vi "fit function - hyperbola.vi"(3 "output control":T1, 4 "data":T2, 5 "X":dbl[](array[numeric]), 6 "a":dbl[](array[numeric])) -> (0 "error out":errorcluster, 1 "f'(X,a)":dbl[][](array[numeric]), 2 "f(X,a)":dbl[](array[numeric]))   [LabVIEW 2018]
doc: "This template is the starting point for creating a model function to be passed to the Nonlinear Curve Fit.vi."
uses:
  <vilib>/gmath/NumericalOptimization/objective function data.ctl
  <vilib>/gmath/NumericalOptimization/LM_output select.ctl
  <vilib>/gmath/NI_Gmath.lvlib
panel:
  in  "fit":enum16{"other", "3par", "5par"}(ring)=enum."3par"
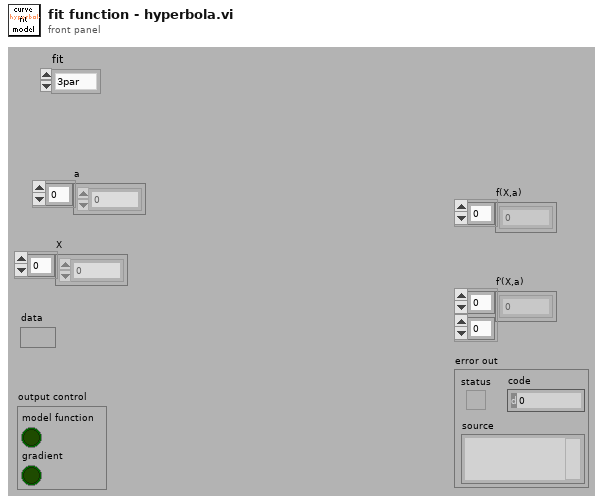
[diagram p1: front panel]
types:
  T1 = typedef "NI_Gmath.lvlib/LM_output select.ctl" = cluster{"model function":bool, "gradient":bool}
  T2 = typedef "NI_Gmath.lvlib/objective function data.ctl" = variant
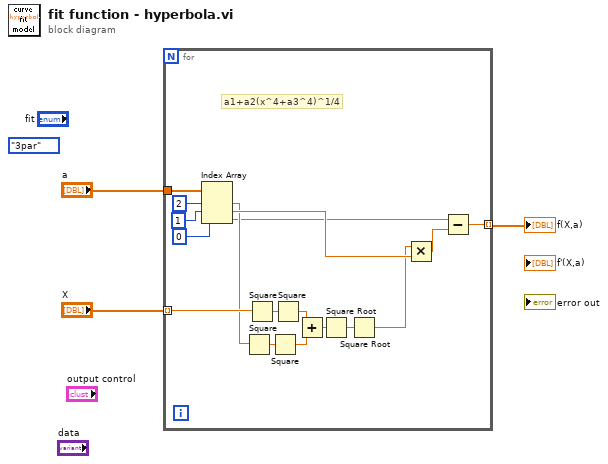
[diagram p0: block diagram]
diagram:
  (unwired) enum16{"other", "3par", "5par"}."3par" ("action")
  n1 = for {
    tunnel: "a" -> [w20]
    tunnel: "X" -> [w18] mode=indexing
    tunnel: [w19] -> w1 mode=indexing
    # "a1+a2(x^4+a3^4)^1/4"
    n2 = Index Array(array=w20, index #1=2 ("index"), index #2=1 ("index"), index #3=0 ("index")) -> (element #1=w11:dbl, element #2=w14:dbl, element #3=w7:dbl)
    n3 = Square(x=w11) -> (x^2=w12:dbl)
    n4 = Square(x=w18) -> (x^2=w13:dbl)
    n5 = Square(x=w12) -> (x^2=w9:dbl)
    n6 = Square(x=w13) -> (x^2=w10:dbl)
    n7 = Add(x=w10, y=w9) -> (x+y=w6:dbl)
    n8 = Square Root(x=w6) -> (sqrt(x)=w5:dbl)
    n9 = Square Root(x=w5) -> (sqrt(x)=w4:dbl)
    n10 = Multiply(x=w4, y=w14) -> (x*y=w8:dbl)
    n11 = Subtract(x=w7, y=w8) -> (x-y=w19:dbl)
  }
  "f(X,a)" <- w1
